vi "perform.vi"(8 "error in (no error)":errorcluster, 10 "Sensor Data":T2 {"Robot Heading" format="%05.1f"; "Wind Direction" format="%05.1f"}, 11 "Drive in":refnum<class "Drive.lvclass">) -> (0 "error out":errorcluster, 2 "Desired Location":T1, 3 "Drive out":refnum<class "Drive.lvclass">)   [LabVIEW 2011, in "Drive.lvclass"]
uses:
  Drive.lvclass
  2-RIO/2 Typedefs/sensorData.ctl
  2-RIO/2 Typedefs/UTM Location.ctl
  2-RIO/2 Typedefs/heading.ctl
  Drive.lvclass/Drive.ctl
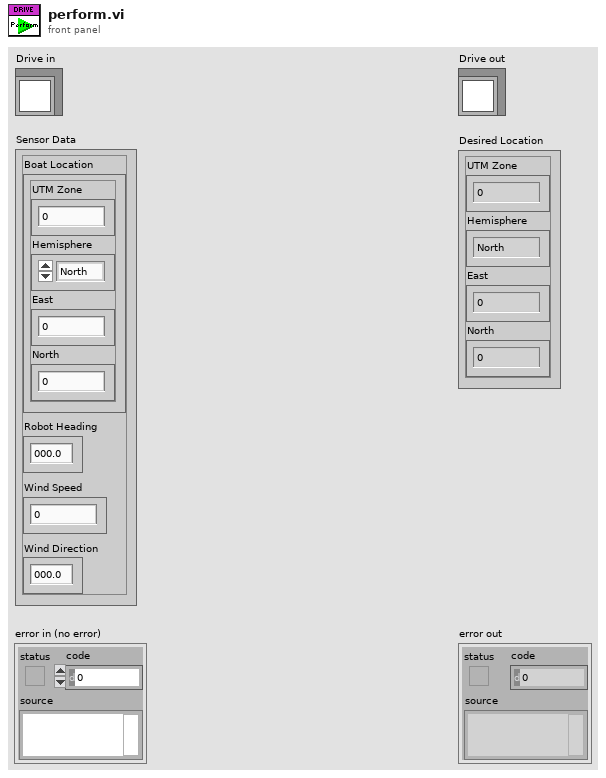
[diagram p1: front panel]
types:
  T1 = typedef "UTM Location.ctl" = cluster{"UTM Zone":dbl, "Hemisphere":enum16{"North", "South"}, "East":dbl, "North":dbl}
  T2 = typedef "sensorData.ctl" = cluster{"Boat Location":T1, "Robot Heading ":T3, "Wind Speed":dbl, "Wind Direction":T3}
  T3 = typedef "heading.ctl" = dbl
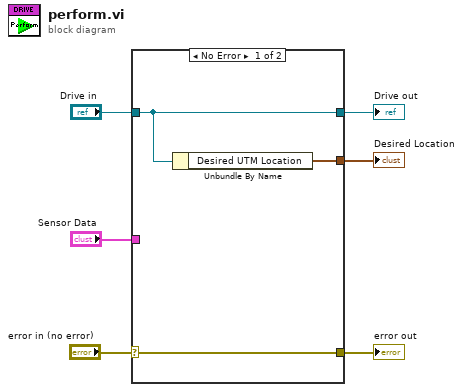
[diagram p0: block diagram]
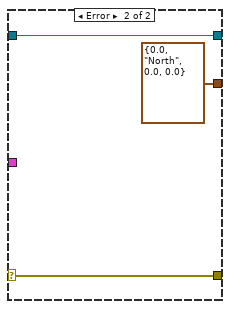
[diagram p2: hidden frame]
diagram:
  n1 = case shown="No Error" "error in (no error)" {
    selector: "error in (no error)" -> [w9 w11]
    tunnel: [w9 w11] -> w5
    tunnel: "Drive in" -> [w8 w12]
    tunnel: [w8 w12] -> w3
    tunnel: "Sensor Data" -> [_ _]
    tunnel: [w7 T1 {"UTM Zone"=0.0, "Hemisphere"=enum."North", "East"=0.0, "North"=0.0} ("Desired UTM Location")] -> w1
    frame No Error {
      n2 = Unbundle By Name(w8) -> ("Desired UTM Location"=w7:T1)
    }
    frame Error {
    }
  }
  "error out" <- w5
  "Drive out" <- w3
  "Desired Location" <- w1
